vi "InsertMoney.vi"(3 "Error In":errorcluster) -> (0 "Error Out":errorcluster, 1 "InsertMoney":string=" 0", 2 "InsertsMoney":i32)   [LabVIEW 2020]
doc: "This VI is dialog program to simulate process of accepcting money by vending machine. Comments in Polish."
uses:
  Ctrls/1zl.ctl
  Ctrls/2zl.ctl
  Ctrls/5zl.ctl
panel:
  in  "5":T1
  in  "Stop":bool
  in  "2":T2
  in  "1":T3
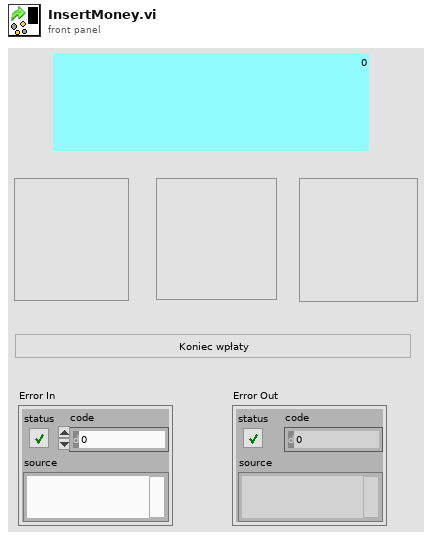
[diagram p1: front panel]
types:
  T1 = typedef "5zl.ctl" = bool
  T2 = typedef "2zl.ctl" = bool
  T3 = typedef "1zl.ctl" = bool
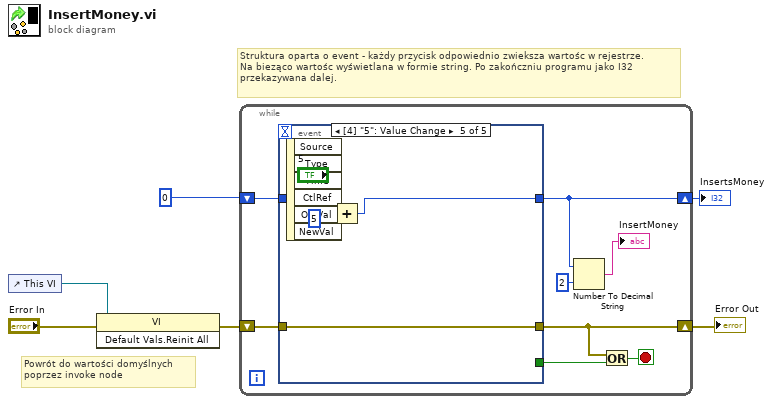
[diagram p0: block diagram]
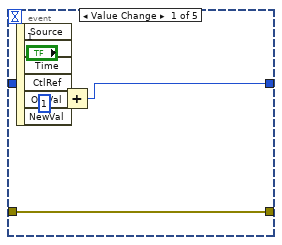
[diagram p2: hidden frame]
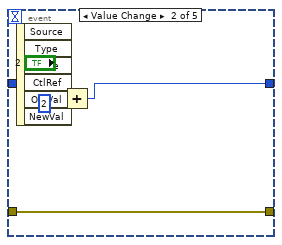
[diagram p3: hidden frame]
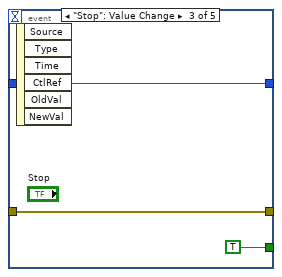
[diagram p4: hidden frame]
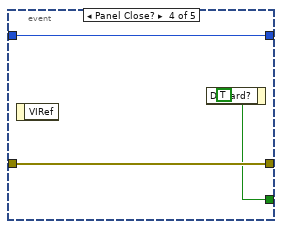
[diagram p5: hidden frame]
diagram:
  # "Struktura oparta o event - każdy przycisk odpowiednio zwieksza wartośc w rejestrze.\nNa bieząco wartośc wyświetlana w formie string. Po zakończniu programu jako I32\nprzekazywana dalej."
  # "Powrót do wartości domyślnych\npoprzez invoke node"
  n1 = control-ref of="This VI"() -> (w1:refnum<vi>)
  n2 = invoke class="VI" method="Default Vals.Reinit All"(reference=w1, error in="Error In") -> (error out=w2:errorcluster)  [unwired: 1 in, 2 out]
  n3 = while {
    shift-right: [w13] -> w5
    shift-left: w2 -> [w14]
    shift-right: [w7] -> w3
    shift-left: 0 -> [w9]
    stop <- w12 stop-if-true
    n4 = event shown="[4] \"5\": Value Change" {
      selector: _ -> [_ _ _ _ _]
      dyn-events: _ -> [_ _ _ _ _]
      timeout: _ -> [_ _ _ _ _]
      tunnel: w14 -> [w18 w22 w25 w28 w32]
      tunnel: [w18 w22 w25 w28 w32] -> w13
      tunnel: w9 -> [w17 w21 w24 w27 w31]
      tunnel: [w15 w19 w24 w27 w29] -> w7
      tunnel: [_ _ TRUE w26 _] -> w8
      event Value Change {
        n5 = event-data() -> ()  [unwired: 1 in, 6 out]
        n6 = Add(x=w17, y=1) -> (x+y=w15:i32)
      }
      event Value Change {
        n7 = event-data() -> ()  [unwired: 1 in, 6 out]
        n8 = Add(x=w21, y=2) -> (x+y=w19:i32)
      }
      event "Stop": Value Change {
        n9 = event-data() -> ()  [unwired: 1 in, 6 out]
      }
      event Panel Close? {
        w26 = TRUE
        n10 = event-data() -> ()  [unwired: 1 in, 1 out]
        n11 = event-data("Discard?"=w26) -> ()  [unwired: 1 in, 1 out]
      }
      event Value Change {
        n12 = event-data() -> ()  [unwired: 1 in, 6 out]
        n13 = Add(x=w31, y=5) -> (x+y=w29:i32)
      }
    }
    n14 = Number To Decimal String(number=w7, width (-)=i16 2) -> (decimal integer string=→"InsertMoney":string)
    n15 = Or(x=w13, y=w8) -> (x .or. y?=w12:bool)
  }
  "InsertsMoney" <- w3
  "Error Out" <- w5
